vi "stepper-read.vi"(8 "error in (no error)":errorcluster, 11 "Stepper.lvclass":refnum<class "Stepper.lvclass">) -> (0 "error out":errorcluster, 2 "Result":dbl[](array[numeric]), 3 "Stepper.lvclass Out":refnum<class "Stepper.lvclass">)   [LabVIEW 2018, in "Stepper.lvclass"]
uses:
  Stepper.lvclass
  Users/Shared/github/NHMFL_Core/Libraries/Instruments/Instrument Driver/Instrument Driver.lvclass
  resonant_ultrasound_arxiv/maglab ultrasound -- arkady --arxiv/publisher action.ctl
  NHMFL_Core/Libraries/Instruments/Instrument Driver/Instrument Driver.lvclass/Instrument Driver.ctl
  NHMFL_Core/Libraries/Instruments/Instrument Driver/Write Channel names.vi
  NHMFL_Core/Libraries/Instruments/Instrument Driver/Write Channel units.vi
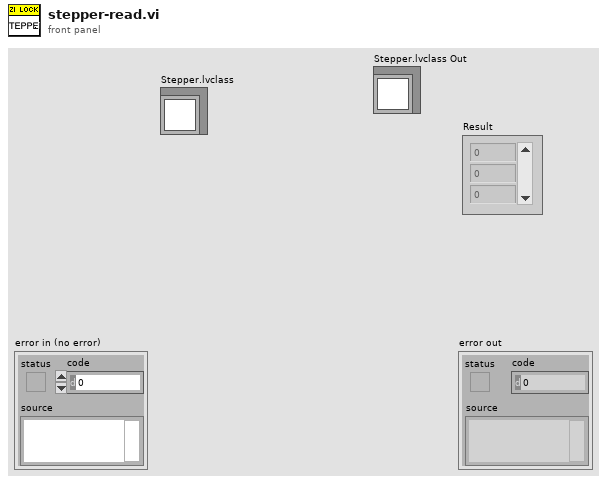
[diagram p1: front panel]
types:
  T1 = typedef "publisher action.ctl" = enum16{"set", "get", "init", "check"}
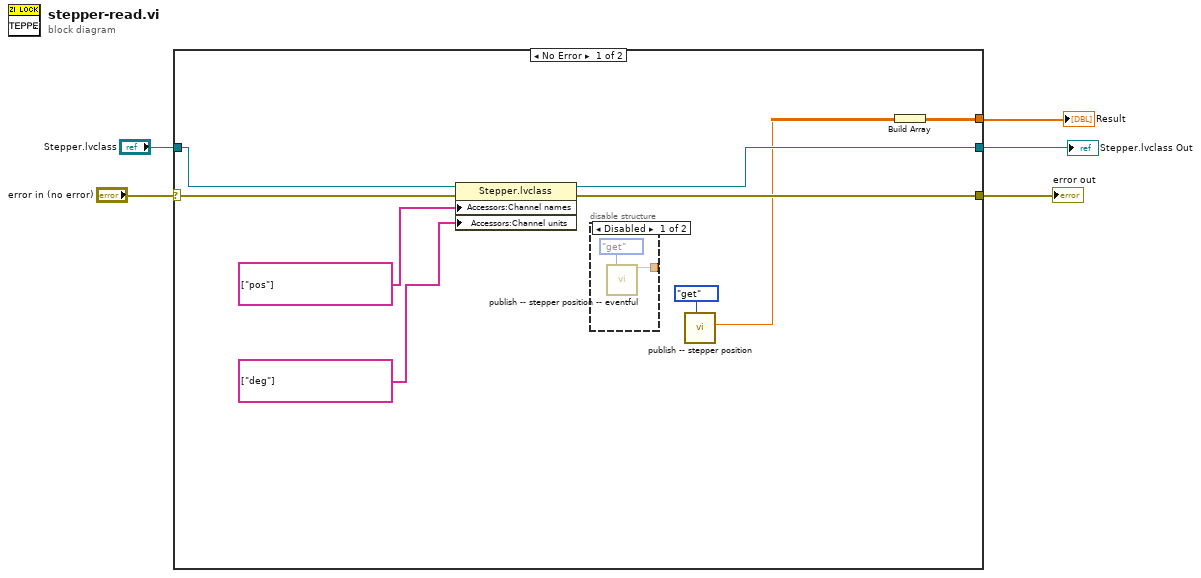
[diagram p0: block diagram]
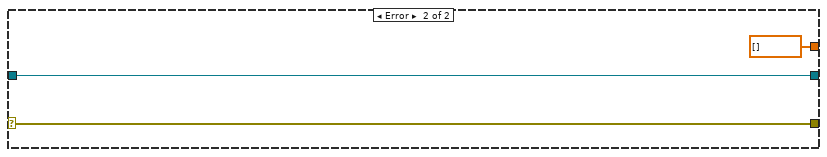
[diagram p3: hidden frame]
diagram:
  n1 = case shown="No Error" "error in (no error)" {
    selector: "error in (no error)" -> [w11 w19]
    tunnel: [w10 w19] -> w4
    tunnel: [w12 w18] -> w2
    tunnel: "Stepper.lvclass" -> [w13 w18]
    tunnel: [w14 dbl[] []] -> w3
    frame No Error {
      n2 = property class="Stepper.lvclass"(reference=w13, error in=w11, "Accessors:Channel names"=string[] ["pos"] ("Channel names"), "Accessors:Channel units"=string[] ["deg"] ("Channel names")) -> (reference out=w12:refnum<class "Stepper.lvclass">, error out=w10:errorcluster)
      n3 = disable-structure shown="Disabled" {
        disable-tunnel: [w15 _] -> _
        frame Disabled {
          n4 = call "publish -- stepper position -- eventful.vi"("publisher action"=publisher_action."get") -> ("step out (Hz)"=w15:dbl)  [unwired: 11 in, 3 out]
        }
        frame Enabled {
        }
      }
      n5 = call "publish -- stepper position.vi"("publisher action"=publisher_action."get") -> ("stepper pos OUT"=w6:dbl)  [unwired: 10 in]
      n6 = Build Array(w6) -> (w14:dbl[])
    }
    frame Error {
    }
  }
  "error out" <- w4
  "Result" <- w3
  "Stepper.lvclass Out" <- w2
